vi "Detect String Encoding.vi"(7 "Strip BOM (T)":bool=TRUE, 8 "error in":errorcluster, 11 "String":string) -> (0 "error out":errorcluster, 2 "Encoding":T1, 3 "String out":string)   [LabVIEW 2020, in "G-Unicode.lvlib"]
doc: "Detect the input string character encoding. If <b>String</b> contains a Byte Order Mark (BOM) and <b>Strip BOM</b> is TRUE, the BOM will be removed from <b>String out</b>. Otherwise the string is unchanged.\n\nThe encoding of the input string is determined based on BOM, statistical tests, and valid UTF-8 encoding ranges. Note that an ASCII string (bytes in range 0-127) will be detected as UTF-8.\n\n<b>Note:</b> This function is not 100% accurate, and can return the incorrect encoding for certain byte orders."
uses:
  G-Unicode.lvlib
  Controls/String Encoding.ctl
  Controls/Detect String Encoding Steps.ctl
  f4e2713d-ca87-487a-b901-d606fc3002c3.vi
  SubVIs/Byte Order Marks.vi
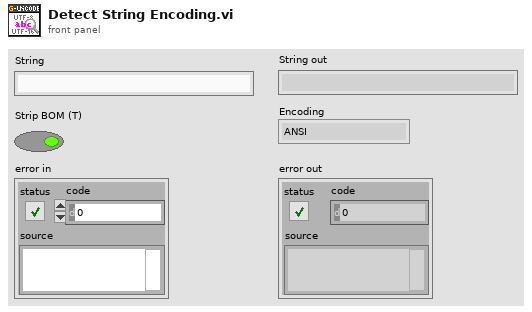
[diagram p1: front panel]
types:
  T1 = typedef "G-Unicode.lvlib/String Encoding.ctl" = enum16{"ANSI", "UTF-8", "UTF-16LE", "UTF-16BE", "Unknown"}
  T2 = typedef "G-Unicode.lvlib/Detect String Encoding Steps.ctl" = enum16{"BOM", "Test UTF-16", "Test UTF-8"}
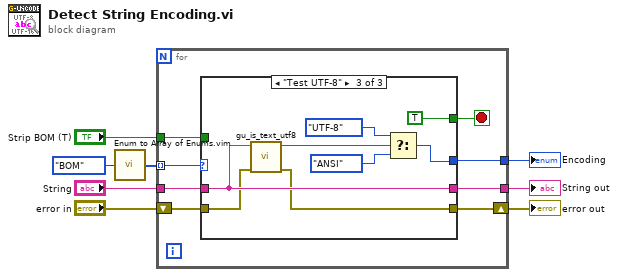
[diagram p0: block diagram]
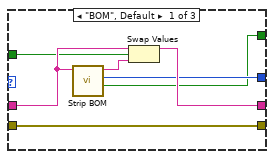
[diagram p2: hidden frame]
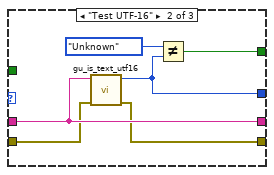
[diagram p3: hidden frame]
diagram:
  n1 = call "Enum to Array of Enums.vim"("enum"=Detect_String_Encoding_Steps."BOM" ("Encoding Checks")) -> ("array of enums"=w8:T2[])
  n2 = for {
    tunnel: w8 -> [w10] mode=indexing
    tunnel: "String" -> [w16]
    tunnel: [w14] -> w6
    tunnel: [w13] -> w5
    shift-right: [w11] -> w3
    shift-left: "error in" -> [w12]
    tunnel: "Strip BOM (T)" -> [w9]
    stop <- w15 stop-if-true
    n3 = case shown="\"Test UTF-8\"" w10 {
      tunnel: w16 -> [w21 w29 w37]
      tunnel: [w17 w26 TRUE ("selection")] -> w15
      tunnel: [w19 w29 w37] -> w14
      tunnel: [w18 w28 w31] -> w13
      tunnel: w12 -> [w23 w25 w36]
      tunnel: [w23 w24 w35] -> w11
      tunnel: w9 -> [w20 _ _]
      frame "BOM", Default {
        n4 = call "Strip BOM.vi"("String"=w21) -> ("BOM Found"=w17:bool, "Encoding"=w18:T1, "String without BOM"=w22:string)  [unwired: 8 in]
        n5 = Swap Values(12:w21, 13:w20, 14:w22) -> (1:w19:string)  [unwired: 1 out]
      }
      frame "Test UTF-16" {
        n6 = call "gu_is_text_utf16.vi"("error in"=w25, "String"=w29) -> ("error out"=w24:errorcluster, "Encoding"=w28:T1)  [unwired: 8 in]
        n7 = Not Equal?(x=String_Encoding."Unknown" ("y"), y=w28) -> (x != y?=w26:bool)
      }
      frame "Test UTF-8" {
        n8 = call "gu_is_text_utf8.vi"("error in"=w36, "Encoded String"=w37) -> ("error out"=w35:errorcluster, "UTF-8"=w33:bool)  [unwired: 8 in]
        n9 = Select(t=String_Encoding."UTF-8" ("Encoding"), s=w33, f=String_Encoding."ANSI") -> (s? t:f=w31:T1)
      }
    }
  }
  "Encoding" <- w5
  "String out" <- w6
  "error out" <- w3
